vi "ep_Check Record Info Validation.vi"(8 "error in (no error)":errorcluster, 11 "record info in":T1={"station name"="", "recording device name"="", "line frequency [Hz]"=50.0, "timestamp multiplier"=1.0}) -> (0 "error out":errorcluster, 3 "record info out":T1={"station name"="", "recording device name"="", "line frequency [Hz]"=50.0, "timestamp multiplier"=1.0})   [LabVIEW 2011, in "NI_EP_COMTRADE.lvlib"]
uses:
  <vilib>/addons/Electrical Power/File IO/NI_EP_COMTRADE.lvlib
  <vilib>/addons/Electrical Power/File IO/COMTRADE/typedefs/ep_System Record Inf.ctl
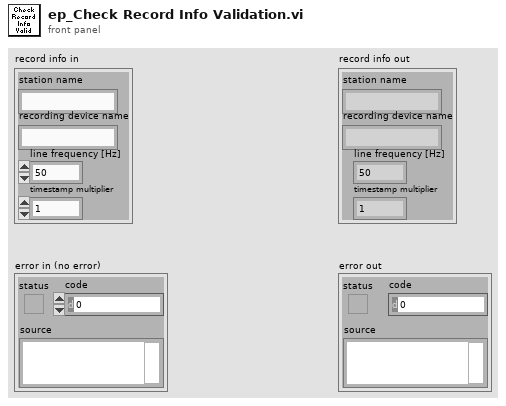
[diagram p1: front panel]
types:
  T1 = typedef "NI_EP_COMTRADE.lvlib/ep_System Record Inf.ctl" = cluster{"station name":string, "recording device name":string, "line frequency [Hz]":sgl, "timestamp multiplier":sgl}
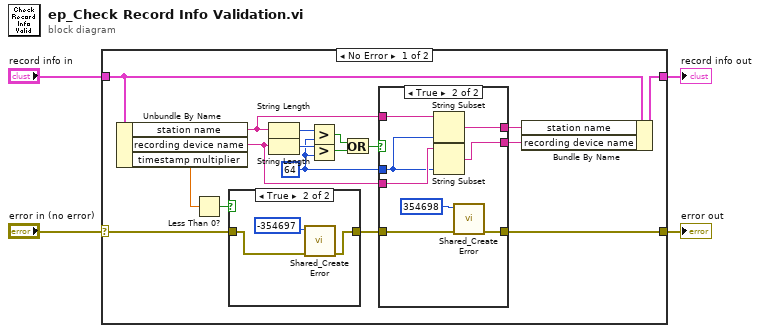
[diagram p0: block diagram]
diagram:
  n1 = case shown="No Error" "error in (no error)" {
    selector: "error in (no error)" -> [w5 w38]
    tunnel: [w9 w38] -> w3
    tunnel: "record info in" -> [w11 w37]
    tunnel: [w12 w37] -> w1
    frame No Error {
      w14 = 64 ("y")
      n2 = Unbundle By Name(w11) -> ("station name"=w16:string, "recording device name"=w15:string, "timestamp multiplier"=w8:sgl)
      n3 = Less Than 0?(x=w8) -> (x < 0?=w7:bool)
      n4 = case shown="True" w7 {
        tunnel: [w22 w23] -> w6
        tunnel: w5 -> [w22 w25]
        frame False {
        }
        frame True {
          n5 = call <vilib>:"Shared_Create Error.vi"("error in (no error)"=w25, "error code (0)"=-354697 ("code")) -> ("error out"=w23:errorcluster)  [unwired: 9 in]
        }
      }
      n6 = String Length(string=w16) -> (length=w21:i32)
      n7 = String Length(string=w15) -> (length=w20:i32)
      n8 = Greater?(x=w21, y=w14) -> (0:w19:bool)
      n9 = Greater?(x=w20, y=w14) -> (0:w18:bool)
      n10 = Or(x=w19, y=w18) -> (x .or. y?=w17:bool)
      n11 = case shown="True" w17 {
        tunnel: w16 -> [w28 w36]
        tunnel: w15 -> [w27 w35]
        tunnel: w14 -> [_ w34]
        tunnel: w6 -> [w26 w31]
        tunnel: [w28 w33] -> w13
        tunnel: [w27 w32] -> w10
        tunnel: [w26 w30] -> w9
        frame False {
        }
        frame True {
          n12 = String Subset(string=w36, length (rest)=w34) -> (substring=w33:string)  [unwired: 1 in]
          n13 = String Subset(string=w35, length (rest)=w34) -> (substring=w32:string)  [unwired: 1 in]
          n14 = call <vilib>:"Shared_Create Error.vi"("error in (no error)"=w31, "error code (0)"=354698 ("code")) -> ("error out"=w30:errorcluster)  [unwired: 9 in]
        }
      }
      n15 = Bundle By Name(cluster=w11, "station name"=w13, "recording device name"=w10) -> (w12:T1)
    }
    frame Error {
    }
  }
  "error out" <- w3
  "record info out" <- w1
